vi "D单元件读写.vi"(8 "错误输入":errorcluster, 9 "Read？":bool, 10 "Component Assemble Input":T1, 11 "引用":refnum<k7>) -> (0 "错误输出":errorcluster, 2 "D Value":i32, 3 "引用输出":refnum<k7>)   [LabVIEW 2017]
uses:
  Component Assemble Input.ctl
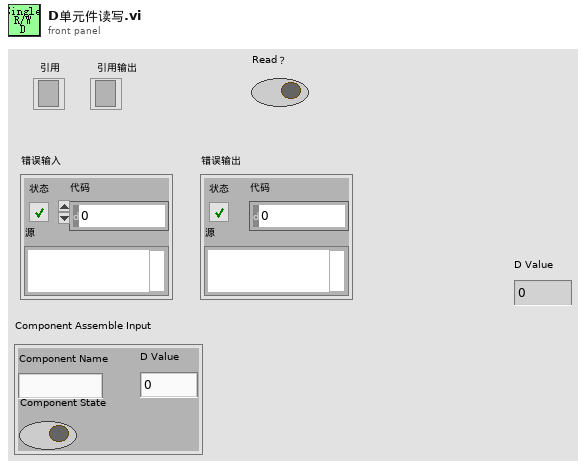
[diagram p1: front panel]
types:
  T1 = typedef "Component Assemble Input.ctl" = cluster{"Component Name":string, "Component State":bool, "D Value":i32}
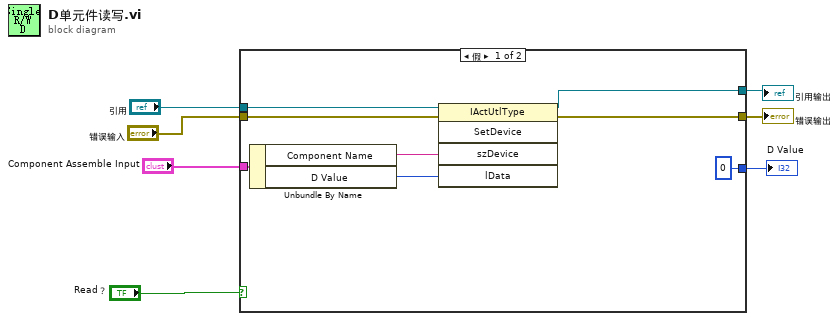
[diagram p0: block diagram]
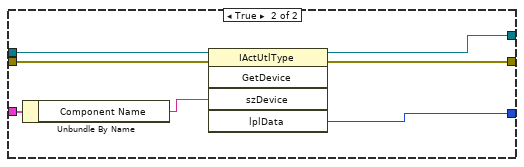
[diagram p2: hidden frame]
diagram:
  n1 = case shown="假" "Read？" {
    tunnel: "引用" -> [w15 w22]
    tunnel: [w11 w21] -> w6
    tunnel: "错误输入" -> [w14 w20]
    tunnel: [w10 w19] -> w4
    tunnel: "Component Assemble Input" -> [w13 w18]
    tunnel: [0 ("lplData") w16] -> w1
    frame False {
      n2 = Unbundle By Name(w13) -> ("Component Name"=w12:string, "D Value"=w8:i32)
      n3 = invoke on="调用节点" class="IActUtlType" method="SetDevice"(reference=w15, error in=w14, "szDevice"=w12, "lData"=w8) -> (reference out=w11:refnum<k7>, error out=w10:errorcluster)  [unwired: 1 in, 3 out]
    }
    frame True {
      n4 = Unbundle By Name(w18) -> ("Component Name"=w17:string)
      n5 = invoke on="调用节点" class="IActUtlType" method="GetDevice"(reference=w22, error in=w20, "szDevice"=w17) -> (reference out=w21:refnum<k7>, error out=w19:errorcluster, "lplData"=w16:i32)  [unwired: 2 in, 2 out]
    }
  }
  "引用输出" <- w6
  "错误输出" <- w4
  "D Value" <- w1
